vi "test.vi"() -> ()   [LabVIEW 2019]
uses:
  mytype.ctl
panel:
  out "indices":i32[](array[numeric])
  in  "Dims":u64[](array[numeric])=[3, 4]
  in  "path":string="test.h5"
  in  "My Type":T1={"My Integer"=1, "My Cluster"={"My Numeric in Cluster"=1.0, "My String in Cluster"="asdf"}, "My Array"=[[1, 1], [1, 1], [1, 1]], "My String"=""}
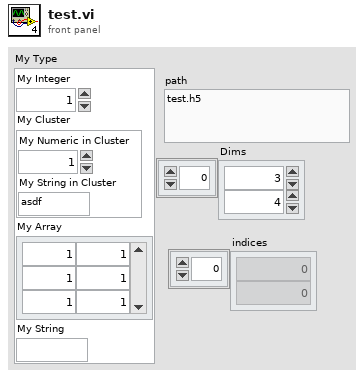
[diagram p1: front panel]
types:
  T1 = typedef "mytype.ctl" = cluster{"My Integer":i32, "My Cluster":cluster{"My Numeric in Cluster":dbl, "My String in Cluster":string}, "My Array":i32[][], "My String":string}
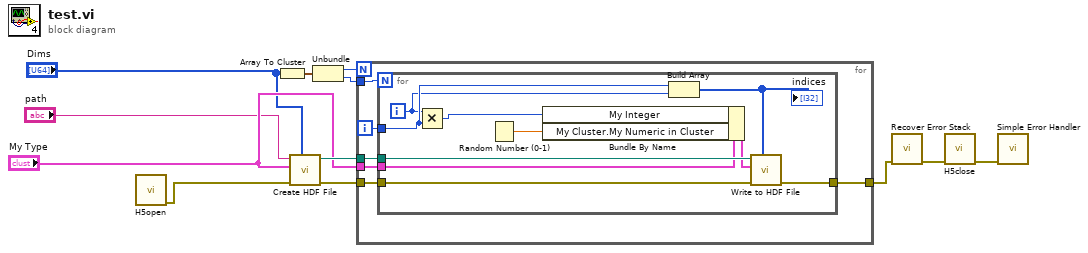
[diagram p0: block diagram]
diagram:
  n1 = call <vilib>:"H5open.vi"() -> ("error out"=w1:errorcluster)  [unwired: 9 in]
  n2 = Array To Cluster(array="Dims") -> (cluster=w8:cluster{"Dims[0]":u64, "Dims[1]":u64})
  n3 = call "Create HDF File.vi"("Dims"="Dims", "error in (no error)"=w1, "My Type"="My Type", "path"="path") -> ("error out"=w10:errorcluster, "path out"=w12:path)  [unwired: 6 in]
  n4 = Unbundle(w8) -> ("Dims[0]"=w7:u64, "Dims[1]"=w6:u64)
  n5 = for {
    N: w7 -> [_]
    tunnel: w12 -> [w18]
    tunnel: "My Type" -> [w17]
    tunnel: w6 -> [w14]
    tunnel: w10 -> [w16]
    tunnel: [w15] -> w4
    i -> [w13]
    n6 = for {
      N: w14 -> [_]
      tunnel: w18 -> [w28]
      tunnel: w17 -> [w27]
      tunnel: w13 -> [w21]
      tunnel: w16 -> [w26]
      tunnel: [w25] -> w15
      i -> [w20]
      n7 = Multiply(x=w20, y=w21) -> (x*y=w23:i32)
      n8 = Random Number (0-1)() -> (number: 0 to 1=w19:dbl)
      n9 = Bundle By Name(cluster=w27, "My Integer"=w23, "My Cluster.My Numeric in Cluster"=w19) -> (w24:T1)
      n10 = Build Array(w21, w20) -> (w22:i32[])
      "indices" <- w22
      n11 = call "Write to HDF File.vi"("indices"=w22, "error in (no error)"=w26, "My Type"=w24, "path"=w28) -> ("error out"=w25:errorcluster)  [unwired: 7 in]
    }
  }
  n12 = call <vilib>:"Recover Error Stack.vi"("error in (no error)"=w4) -> ("error out"=w3:errorcluster)  [unwired: 5 in, 3 out]
  n13 = call <vilib>:"H5close.vi"("error in (no error)"=w3) -> ("error out"=w2:errorcluster)  [unwired: 8 in]
  n14 = call <vilib>:"Simple Error Handler.vi"("error in (no error)"=w2) -> ()  [unwired: 4 in, 5 out]
